vi "KE622x -- Get Questionable Event Enable Reg State.vi"(0 "VISA Resource In":refnum<visa-resource-name>, 1 "Error Query (T)?":bool=TRUE, 11 "error in (no error)":errorcluster) -> (4 "VISA Resource Out (dupl)":refnum<visa-resource-name>, 8 "KE622x Questionable Event Enabled Reg":T1, 15 "error out":errorcluster)   [LabVIEW 2009, in "Keithley 622x.lvlib"]
doc: "Returns the bits in the 'Questionable Event Enable' register of the Status Model. Note that only the used (named) bits are returned."
uses:
  <instrlib>/Keithley 622x LV 2009/Utility/Status Registers/Typedefs/KE622x -- Questionable Event Enable Reg State.ctl
  <instrlib>/Keithley 622x LV 2009/Keithley 622x.lvlib
panel:
  out "Reg Num (dec)":u16 format="%0d"
  out "Reg Num (binary)":u16 format="%016b"
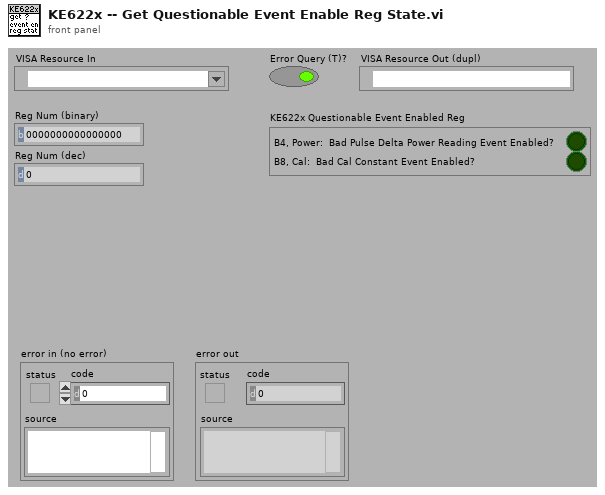
[diagram p1: front panel]
types:
  T1 = typedef "Keithley 622x.lvlib/KE622x -- Questionable Event Enable Reg State.ctl" = cluster{"B4, Power:  Bad Pulse Delta Power Reading Event Enabled?":bool, "B8, Cal:  Bad Cal Constant Event Enabled?":bool}
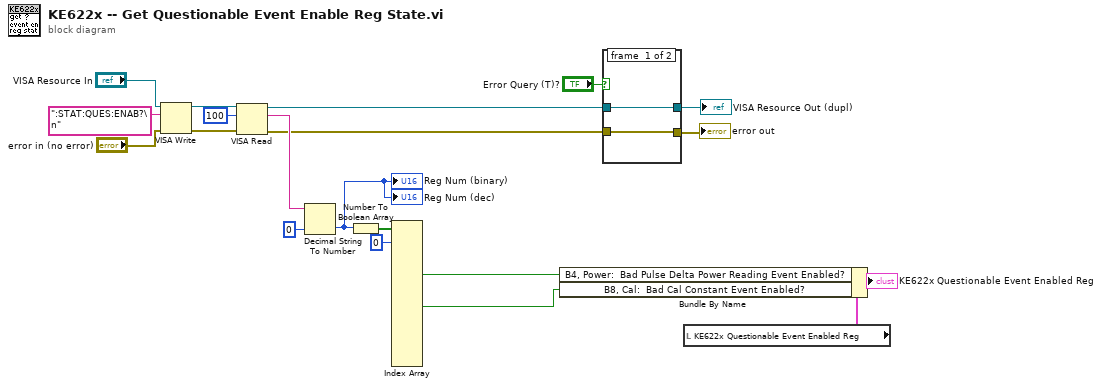
[diagram p0: block diagram]
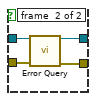
[diagram p2: hidden frame]
diagram:
  n1 = VISA Write(VISA resource name="VISA Resource In", write buffer=":STAT:QUES:ENAB?\n", error in (no error)="error in (no error)") -> (VISA resource name out=w17:refnum<visa-resource-name>, error out=w16:errorcluster)  [unwired: 1 out]
  n2 = VISA Read(VISA resource name=w17, byte count=u32 100, error in (no error)=w16) -> (VISA resource name out=w5:refnum<visa-resource-name>, read buffer=w14:string, error out=w6:errorcluster)  [unwired: 1 out]
  n3 = Decimal String To Number(string=w14, default (0L)=u16 0 ("default (0 I32)")) -> (number=w10:u16)  [unwired: 2 out]
  "Reg Num (binary)" <- w10
  "Reg Num (dec)" <- w10
  n4 = Number To Boolean Array(number=w10) -> (Boolean array=w12:bool[])
  n5 = Index Array(array=w12, index #1=0 ("index")) -> (element #5=w2:bool, element #9=w1:bool)  [unwired: 15 in, 14 out]
  n6 = case shown="True" "Error Query (T)?" {
    tunnel: w6 -> [w21 w26]
    tunnel: w5 -> [w22 w25]
    tunnel: [w21 w24] -> w7
    tunnel: [w22 w23] -> w8
    frame #0 {
    }
    frame #1 {
      n7 = call <instrlib>:"Error Query.vi"("VISA Resource In"=w25, "error in (no error)"=w26) -> ("VISA Resource Out (dupl)"=w23:refnum<visa-resource-name>, "error out"=w24:errorcluster)  [unwired: 10 in, 2 out]
    }
  }
  "VISA Resource Out (dupl)" <- w8
  "error out" <- w7
  n8 = local read "KE622x Questionable Event Enabled Reg"() -> (w11:T1)
  n9 = Bundle By Name(cluster=w11, "B4, Power:  Bad Pulse Delta Power Reading Event Enabled?"=w2, "B8, Cal:  Bad Cal Constant Event Enabled?"=w1) -> (→"KE622x Questionable Event Enabled Reg":T1)
